vi "Backup Database.vi"(6 "progress event":refnum<user-event>, 8 "error in (no error)":errorcluster, 9 "database IDs":cluster{"source":string, "destination":string}={"source"="MAIN", "destination"="MAIN"}, 10 "SQLite3LV Connection dst":refnum<class "sqlite3.lvclass">, 11 "SQLite3LV Connection src":refnum<class "sqlite3.lvclass">) -> (0 "error out":errorcluster, 2 "SQLite3LV Connection out (dst)":refnum<class "sqlite3.lvclass">, 3 "SQLite3LV Connection out (src)":refnum<class "sqlite3.lvclass">)   [LabVIEW 2014, in "SQLite3LV.lvlib" / "sqlite3.lvclass"]
doc: "Initiates a backup of one database to another.\n\nA second active database connection must be supplied to this function.\nRefer to the SQLite3LV Connection documentation for more information regarding backing up databases.\n\nhttps://www.sqlite.org/backup.html\n\nThis VI may be used to backup an in-memory database to a disk-based database.\n\nThe database IDs input controls the name of the source and destination database (default is MAIN)\n\nProgress notifications will be posted to the optionally supplied U8-typed user event. Progress is reported as values ranging from 0 to 100.\n\nThe destination database is automatically locked for the duration of the backup operation.\nThe source database may be locked and unlocked multiple times during the backup operation so that other threads may use the source database connection while the backup operation is in progress."
uses:
  sqlite3.lvclass
  SQLite3LV.lvlib
  sqlite3_64.dll
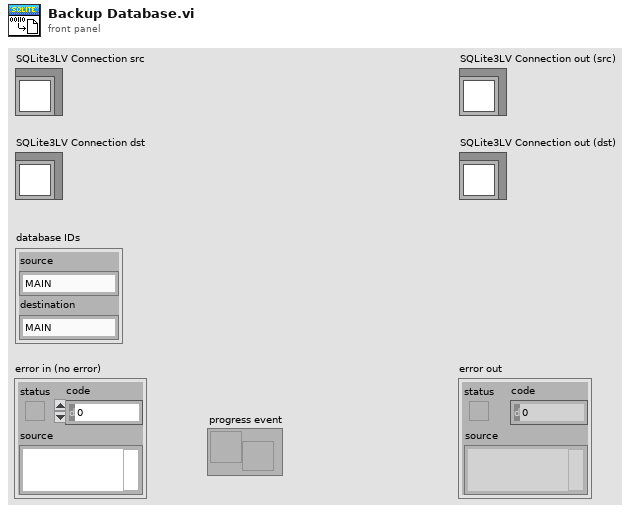
[diagram p1: front panel]
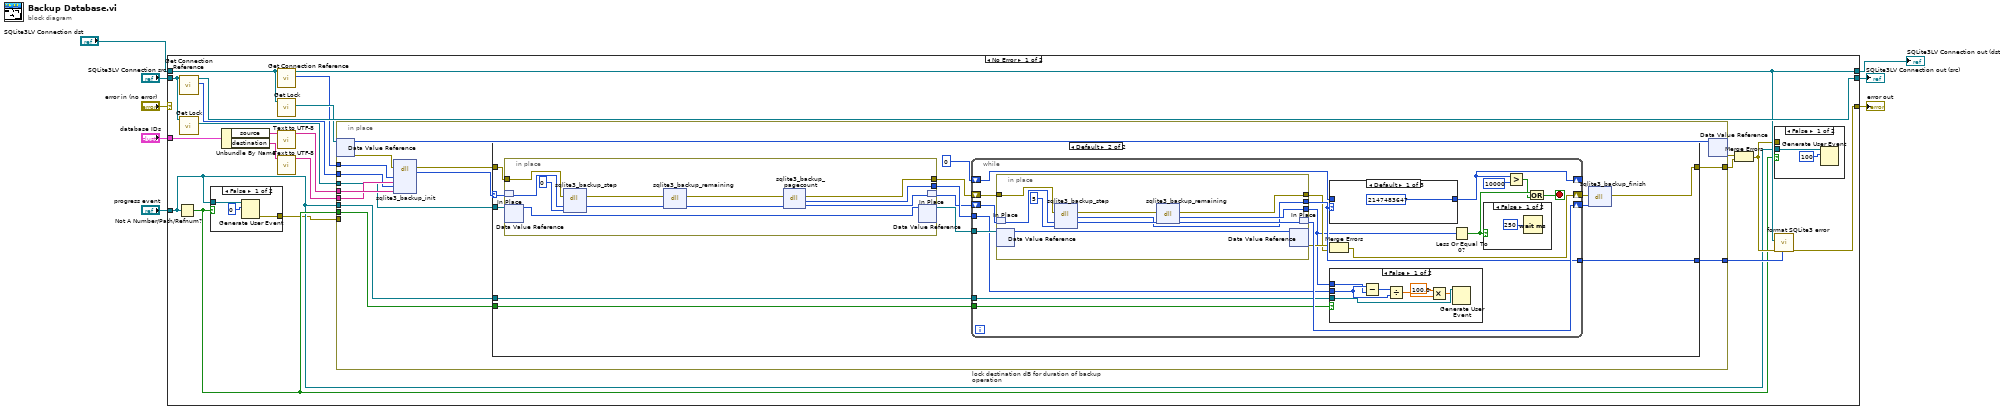
[diagram p0: block diagram]
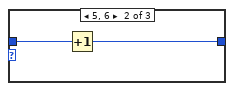
[diagram p6: hidden frame]
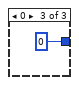
[diagram p7: hidden frame]
diagram:
  n1 = case shown="No Error" "error in (no error)" {
    selector: "error in (no error)" -> [_ w116]
    tunnel: [w15 w116] -> w7
    tunnel: [w29 w115] -> w5
    tunnel: "SQLite3LV Connection src" -> [w28 w115]
    tunnel: "SQLite3LV Connection dst" -> [w27 w114]
    tunnel: [w16 w114] -> w3
    tunnel: "database IDs" -> [w24 _]
    tunnel: "progress event" -> [w10 _]
    frame No Error {
      n2 = Not A Number/Path/Refnum?(number/path/refnum=w10) -> (NaN/Path/Refnum?=w11:bool)
      n3 = call "Get Connection Reference.vi"("SQLite3LV Connection in"=w28) -> ("ppDb"=w19:i64, "SQLite3LV Connection out"=w29:refnum<class "sqlite3.lvclass">)  [unwired: 8 in, 1 out]
      n4 = call "Get Lock.vi"("SQLite3LV Connection in"=w28) -> ("sqlite lock"=w18:refnum<data-value>)  [unwired: 8 in, 2 out]
      n5 = case shown="False" w11 {
        tunnel: w10 -> [w32 _]
        tunnel: [w30 _] -> w9
        frame False {
          n6 = Generate User Event(user event=w32, event data cluster=u8 0 ("x")) -> (error out=w30:errorcluster)  [unwired: 2 in, 1 out]
        }
        frame True {
        }
      }
      n7 = Unbundle By Name(w24) -> ("source"=w22:string, "destination"=w23:string)
      n8 = call "Get Connection Reference.vi"("SQLite3LV Connection in"=w27) -> ("ppDb"=w25:i64, "SQLite3LV Connection out"=w16:refnum<class "sqlite3.lvclass">)  [unwired: 8 in, 1 out]
      n9 = call "Get Lock.vi"("SQLite3LV Connection in"=w27) -> ("sqlite lock"=w26:refnum<data-value>)  [unwired: 8 in, 2 out]
      n10 = call "Text to UTF-8.vi"("text"=w22) -> ("utf-8 text"=w21:string)  [unwired: 9 in, 1 out]
      n11 = call "Text to UTF-8.vi"("text"=w23) -> ("utf-8 text"=w20:string)  [unwired: 9 in, 1 out]
      n12 = in-place "lock destination dB for duration of backup operation" {
        in-place-border: w25 -> [w46]
        in-place-border: w21 -> [w45]
        in-place-border: w20 -> [w44]
        in-place-border: w19 -> [w43]
        in-place-border: w18 -> [w39]
        in-place-border: [w38] -> w17
        in-place-border: [w37] -> w13
        in-place-border: w10 -> [w36]
        in-place-border: w11 -> [w35]
        in-place-border: w9 -> [_]
        n13 = in-place-dvr #1(w26) -> (w47:i32, w41:errorcluster)
        n14 = dll-call lib="C:/Users/BobUser/Desktop/LVTables/sqlite3**.*" fn="sqlite3_backup_init"(error in=w41, "ppDest"=w46, "zDestName"=w44, "ppSourceDb"=w43, "zSourceName"=w45) -> (error out=w40:errorcluster, "psqlite3_backup"=w42:i64)  [unwired: 6 in, 1 out]
        n15 = case shown="Default" w42 {
          selector: w42 -> [_ w60]
          tunnel: w40 -> [w48 w62]
          tunnel: w39 -> [_ w61]
          tunnel: [_ w54] -> w38
          tunnel: [w48 w51] -> w37
          tunnel: w36 -> [_ w50]
          tunnel: w35 -> [_ w49]
          frame 0 {
          }
          frame Default {
            n16 = in-place {
              in-place-border: w62 -> [w113]
              in-place-border: [w103] -> w58
              in-place-border: [w104] -> w53
              n17 = in-place-match #2(w60) -> (w108:i64)
              n18 = in-place-dvr #3(w61) -> (w111:i32)  [unwired: 1 out]
              n19 = dll-call lib="C:/Users/BobUser/Desktop/LVTables/sqlite3**.*" fn="sqlite3_backup_step"(error in=w113, "pp_sqlite3_backup"=w108, "nPage"=0) -> (error out=w105:errorcluster, "pp_sqlite3_backup"=w110:i64)  [unwired: 4 in, 1 out]
              n20 = dll-call lib="C:/Users/BobUser/Desktop/LVTables/sqlite3**.*" fn="sqlite3_backup_remaining"(error in=w105, "pp_sqlite3_backup"=w110) -> (error out=w106:errorcluster, "pp_sqlite3_backup"=w109:i64)  [unwired: 3 in, 1 out]
              n21 = dll-call lib="C:/Users/BobUser/Desktop/LVTables/sqlite3**.*" fn="sqlite3_backup_pagecount"(error in=w106, "pp_sqlite3_backup"=w109) -> (error out=w104:errorcluster, "result"=w103:i32, "pp_sqlite3_backup"=w107:i64)  [unwired: 2 in, 1 out]
              n22 = in-place-dvr #3(w111) -> (w59:refnum<data-value>)  [unwired: 1 out]
              n23 = in-place-match #2(w107) -> (w57:i64)
            }
            n24 = while {
              tunnel: w59 -> [w80]
              tunnel: w58 -> [w64]
              shift-right: [w78] -> w56
              shift-left: w57 -> [w79]
              shift-right: [w75] -> _
              shift-left: 0 ("nPage") -> [w76]
              tunnel: [w71] -> w54
              shift-right: [w67] -> w52
              shift-left: w53 -> [w70]
              tunnel: w50 -> [w66]
              tunnel: w49 -> [w63]
              stop <- w73 stop-if-true
              n25 = in-place {
                in-place-border: [w98] -> w65
                in-place-border: [w95] -> w71
                in-place-border: w70 -> [w94]
                in-place-border: [w93] -> w68
                n26 = in-place-match #4(w79) -> (w99:i64)
                n27 = in-place-dvr #5(w80) -> (w101:i32)  [unwired: 1 out]
                n28 = dll-call lib="C:/Users/BobUser/Desktop/LVTables/sqlite3**.*" fn="sqlite3_backup_step"(error in=w94, "pp_sqlite3_backup"=w99, "nPage"=5) -> (error out=w96:errorcluster, "result"=w95:i32, "pp_sqlite3_backup"=w100:i64)  [unwired: 3 in, 1 out]
                n29 = dll-call lib="C:/Users/BobUser/Desktop/LVTables/sqlite3**.*" fn="sqlite3_backup_remaining"(error in=w96, "pp_sqlite3_backup"=w100) -> (error out=w93:errorcluster, "result"=w98:i32, "pp_sqlite3_backup"=w97:i64)  [unwired: 2 in, 1 out]
                n30 = in-place-dvr #5(w101) -> (w69:errorcluster)  [unwired: 1 out]
                n31 = in-place-match #4(w97) -> (w78:i64)
              }
              n32 = case shown="Default" w71 {
                tunnel: w76 -> [_ w90 _]
                tunnel: [2147483647 w89 0] -> w75
                frame Default {
                }
                frame 5, 6 {
                  n33 = Increment(x=w90) -> (x+1=w89:i32)
                }
                frame 0 {
                }
              }
              n34 = Merge Errors(w69, w68) -> (w67:errorcluster)
              n35 = case shown="False" w63 {
                tunnel: w66 -> [w87 _]
                tunnel: w64 -> [w86 _]
                tunnel: w65 -> [w85 _]
                frame False {
                  n36 = Subtract(x=w86, y=w85) -> (x-y=w84:i32)
                  n37 = Divide(x=w84, y=w86) -> (x/y=w83:dbl)
                  n38 = Multiply(x=100.0, y=w83) -> (x*y=w81:dbl)
                  n39 = Generate User Event(user event=w87, event data cluster=w81) -> ()  [unwired: 2 in, 2 out]
                }
                frame True {
                }
              }
              n40 = Less Or Equal To 0?(x=w65) -> (x <= 0?=w77:bool)
              n41 = case shown="False" w77 {
                frame False {
                  n42 = Wait (ms)(milliseconds to wait=u32 250) -> ()  [unwired: 1 out]
                }
                frame True {
                }
              }
              n43 = Greater?(x=w75, y=10000) -> (0:w72:bool)
              n44 = Or(x=w77, y=w72) -> (x .or. y?=w73:bool)
            }
            n45 = dll-call lib="C:/Users/BobUser/Desktop/LVTables/sqlite3**.*" fn="sqlite3_backup_finish"(error in=w52, "pp_sqlite3_backup"=w56) -> (error out=w51:errorcluster)  [unwired: 4 in, 1 out]
          }
        }
        n46 = in-place-dvr #1(w47) -> (w14:errorcluster)  [unwired: 1 out]
      }
      n47 = Merge Errors(w14, w13) -> (w12:errorcluster)
      n48 = case shown="False" w11 {
        tunnel: w10 -> [w34 _]
        tunnel: w12 -> [_ _]
        frame False {
          n49 = Generate User Event(user event=w34, event data cluster=u8 100 ("x")) -> ()  [unwired: 2 in, 2 out]
        }
        frame True {
        }
      }
      n50 = call "format SQLite3 error.vi"("SQLite3LV Connection result"=w17, "error in (no error)"=w12, "psqlite"=w16) -> ("error out"=w15:errorcluster)  [unwired: 8 in]
    }
    frame Error {
    }
  }
  "error out" <- w7
  "SQLite3LV Connection out (src)" <- w5
  "SQLite3LV Connection out (dst)" <- w3
